vi "Switch Cal Standard.vi"(0 "Cal Standard Sim in":refnum<class "Cal Standard Sim.lvclass">, 5 "Standard Type":T1, 7 "Path Name":string, 11 "error in (no error)":errorcluster) -> (4 "Cal Standard Sim out":refnum<class "Cal Standard Sim.lvclass">, 15 "error out":errorcluster)   [LabVIEW 2023, in "RFFixtureCharact.Instruments.lvlib" / "Cal Standard Sim.lvclass"]
uses:
  Cal Standard Sim.lvclass
  C:/srd-semi-rfcal-software/AuxTools/STSRFFixtureCharactUtility/Source/Code Modules/Fixture/Instruments/Cal Standard/Cal Standard Base/Cal Standard Base.lvclass
  Type Definitions/Standard Type.ctl
  Cal Standard Base/Cal Standard Base.lvclass/Cal Standard Base.ctl
  Cal Standard Base/Properties/Read Instrument Info.vi
  Common/RFCalAndFixtureCharact.Common.lvlib
  RFFixtureCharact.Instruments.lvlib
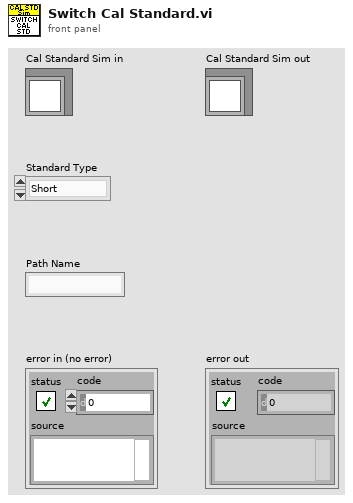
[diagram p1: front panel]
types:
  T1 = typedef "RFFixtureCharact.Instruments.lvlib/Standard Type.ctl" = enum16{"Short", "Open", "Load"}
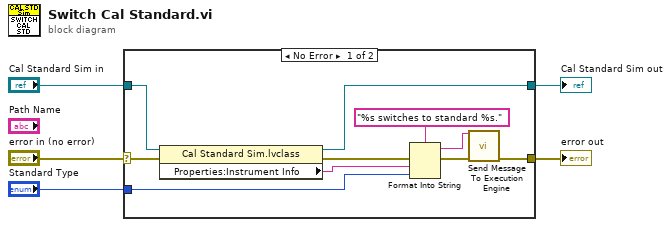
[diagram p0: block diagram]
diagram:
  n1 = case shown="No Error" "error in (no error)" {
    selector: "error in (no error)" -> [w11 w17]
    tunnel: [w15 w17] -> w2
    tunnel: [w8 w16] -> w4
    tunnel: "Cal Standard Sim in" -> [w10 w16]
    tunnel: "Standard Type" -> [w6 _]
    frame No Error {
      n2 = property class="Cal Standard Sim.lvclass"(reference=w10, error in=w11) -> (reference out=w8:refnum<class "Cal Standard Sim.lvclass">, error out=w9:errorcluster, "Properties:Instrument Info"=w7:string)
      n3 = Format Into String(format string="%s switches to standard %s." ("message"), error in=w9, w7, w6) -> (resulting string=w12:string, error out=w14:errorcluster)  [unwired: 1 in]
      n4 = call "Send Message To Execution Engine.vi"("Message"=w12, "error in (no error)"=w14) -> ("error out"=w15:errorcluster)  [unwired: 13 in]
    }
    frame Error {
    }
  }
  "error out" <- w2
  "Cal Standard Sim out" <- w4
